vi "Write Forecast and Price Data to Optimization.vi"(6 "Max Forecast Length (-1: no limit)":i32=-1, 7 "Bus by ID":T1[](array[typedef]), 8 "error in":errorcluster, 11 "Generic Optimization in":refnum<class "Generic Optimization.lvclass">) -> (0 "error out":errorcluster, 3 "Generic Optimization out":refnum<class "Generic Optimization.lvclass">)   [LabVIEW 2018, in "Generic Optimization Actor.lvlib" / "Generic Optimization.lvclass"]
uses:
  Generic Optimization.lvclass
  C:/Users/Administrator/Desktop/2018LabVIEW EMS/EMS Generic Actor/EMS Generic/EMS Generic.lvclass
  C:/Users/Administrator/Desktop/2018LabVIEW EMS/Device Communication and Control Abstract Actor/Device Communication and Control Abstract/Device Communication and Control Abstract.lvclass
  Optimization Controls/Bus by ID.ctl
  <vilib>/ORNL/CSEISMIC DDS/CSEISMIC DDS Base/Data Types/Controls/DeviceID.ctl
  EMS Generic Actor/EMS Generic/EMS Generic.lvclass/EMS Generic.ctl
  <vilib>/ORNL/CSEISMIC DDS/CSEISMIC DDS Base/Data Types/Controls/DeviceClass Selector.ctl
  <vilib>/ORNL/CSEISMIC DDS/CSEISMIC DDS Base/Data Types/DER_Info.ctl
  <vilib>/ORNL/CSEISMIC DDS/CSEISMIC DDS Base/Data Types/SmartRelay_Measurement.ctl
  <vilib>/ORNL/CSEISMIC DDS/CSEISMIC DDS Base/Data Types/DER_Measurement.ctl
  <vilib>/ORNL/CSEISMIC DDS/CSEISMIC DDS Base/Data Types/ForecastData_Data.ctl
  <vilib>/ActorFramework/Actor/Actor.lvclass/Actor.ctl
  Device Communication and Control Abstract Actor/Device Communication and Control Abstract/Device Communication and Control Abstract.lvclass/Device Communication and Control Abstract.ctl
  Device Communication and Control Abstract Actor/Device Communication and Control Abstract Messages/Set ForecastData Long Msg/Set ForecastData Long Msg.lvclass/Set ForecastData Long Msg.ctl
  <vilib>/ActorFramework/Message Enqueuer/Message Enqueuer.lvclass/Message Enqueuer.ctl
  Generic Optimization.lvclass/Generic Optimization.ctl
  Device Communication and Control Abstract Actor/Device Communication and Control Abstract Messages/Set ForecastData Long Msg/Send Set ForecastData Long.vi
  <vilib>/ActorFramework/Actor/Read Caller Enqueuer.vi
  <vilib>/ActorFramework/Message Enqueuer/Enqueue.vi
  Device Communication and Control Abstract Actor/Device Communication and Control Abstract/Device Communication and Control Abstract.lvclass
  C:/Program Files (x86)/National Instruments/LabVIEW 2018/vi.lib/ActorFramework/Actor/Actor.lvclass
  Device Communication and Control Abstract Actor/Device Communication and Control Abstract Messages/Set ForecastData Long Msg/Set ForecastData Long Msg.lvclass
  C:/Program Files (x86)/National Instruments/LabVIEW 2018/vi.lib/ActorFramework/Message/Message.lvclass
  <vilib>/ActorFramework/Message Priority Queue/Priority Enqueue.vi
  <vilib>/ORNL/CSEISMIC DDS/CSEISMIC DDS Base/CSEISMIC DDS.lvclass
  EMS Generic Actor/EMS Generic/EMS Generic.lvclass
  Utilities/Status Messaging.llb/Status Messaging.lvlib
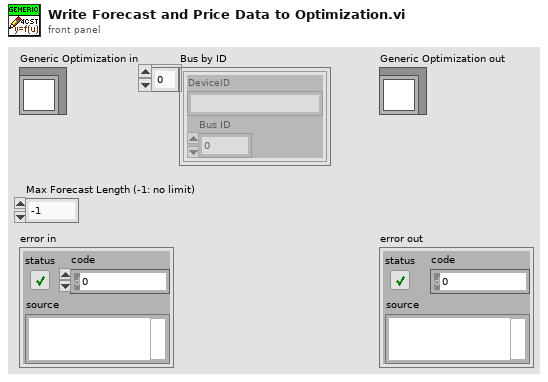
[diagram p1: front panel]
types:
  T1 = typedef "Generic Optimization Actor.lvlib/Generic Optimization.lvclass/Bus by ID.ctl" = cluster{"DeviceID":T2, "Bus ID":dbl}
  T2 = typedef "CSEISMIC DDS.lvlib/CSEISMIC DDS.lvclass/DeviceID.ctl" = string
  T3 = typedef "CSEISMIC DDS.lvlib/CSEISMIC DDS.lvclass/DER_Info.ctl" = cluster{"DeviceID":T2, "LineConfig":u8[], "NominalVoltage(V)":dbl, "PowerRating(kVA)":dbl, "VFControl":bool, "PControl":bool, "QControl":bool, "PFControl":bool, "PVControl":bool, "Droop":bool, "DroopConfigurable":bool, "Unbalanced":bool}
  T4 = typedef "CSEISMIC DDS.lvlib/CSEISMIC DDS.lvclass/ForecastData_Data.ctl" = cluster{"DeviceID":T2, "TargetID":T2, "t0":dbl, "dt":dbl, "Magnitude":dbl[]}
  T5 = typedef "CSEISMIC DDS.lvlib/CSEISMIC DDS.lvclass/SmartRelay_Measurement.ctl" = cluster{"DeviceID":T2, "PrimaryVoltage":dbl[], "SecondaryVoltage":dbl[], "Current":dbl[], "RealPower":dbl[], "ReactivePower":dbl[], "LineConfig":u8[], "Frequency":dbl}
  T6 = typedef "CSEISMIC DDS.lvlib/CSEISMIC DDS.lvclass/DER_Measurement.ctl" = cluster{"DeviceID":T2, "Voltage":dbl[], "Current":dbl[], "RealPower":dbl[], "ReactivePower":dbl[], "LineConfig":u8[], "Frequency":dbl}
  T7 = typedef "EMS Generic Actor.lvlib/EMS Generic.lvclass/Data Type DVRs.ctl" = cluster{"IED_Status":refnum<data-value>, "IED_Status_0":refnum<data-value>, "DER_Measurement":refnum<data-value>, "DER_Info":refnum<data-value>, "DER_Status":refnum<data-value>, "ES_Measurement":refnum<data-value>, "ES_Info":refnum<data-value>, "PV_Info":refnum<data-value>, "SmartRelay_Info":refnum<data-value>, "SmartRelay_Measurement":refnum<data-value>, "Meter_Info":refnum<data-value>, "Meter_Measurement":refnum<data-value>, "HVAC_Status":refnum<data-value>, "HVAC_Measurement":refnum<data-value>, "PriceData_RealTime":refnum<data-value>, "PriceData_Demand":refnum<data-value>, "PriceData_Energy":refnum<data-value>, "ForecastData_Long":refnum<data-value>, "ForecastData_Short":refnum<data-value>, "DER_Control":refnum<data-value>, "DER_SetPointF":refnum<data-value>, "DER_SetPointP":refnum<data-value>, "DER_SetPointQ":refnum<data-value>, "DER_SetPointPF":refnum<data-value>, "DER_SetPointV":refnum<data-value>, "PV_setCurtailment":refnum<data-value>, "PV_setRampRate":refnum<data-value>, "Relay_Control":refnum<data-value>, "Load_Control":refnum<data-value>, "HVAC_Control":refnum<data-value>, "Generator_Info":refnum<data-value>, "ForecastData_Long_Backup":refnum<data-value>, "PriceData_RealTime_Backup":refnum<data-value>}
  T8 = typedef "CSEISMIC DDS.lvlib/CSEISMIC DDS.lvclass/DeviceClass Selector.ctl" = u16
  T9 = typedef "CSEISMIC DDS.lvlib/CSEISMIC DDS.lvclass/PriceData_RealTime.ctl" = cluster{"DeviceID":T2, "t0":dbl, "dt":dbl, "Price":dbl[]}
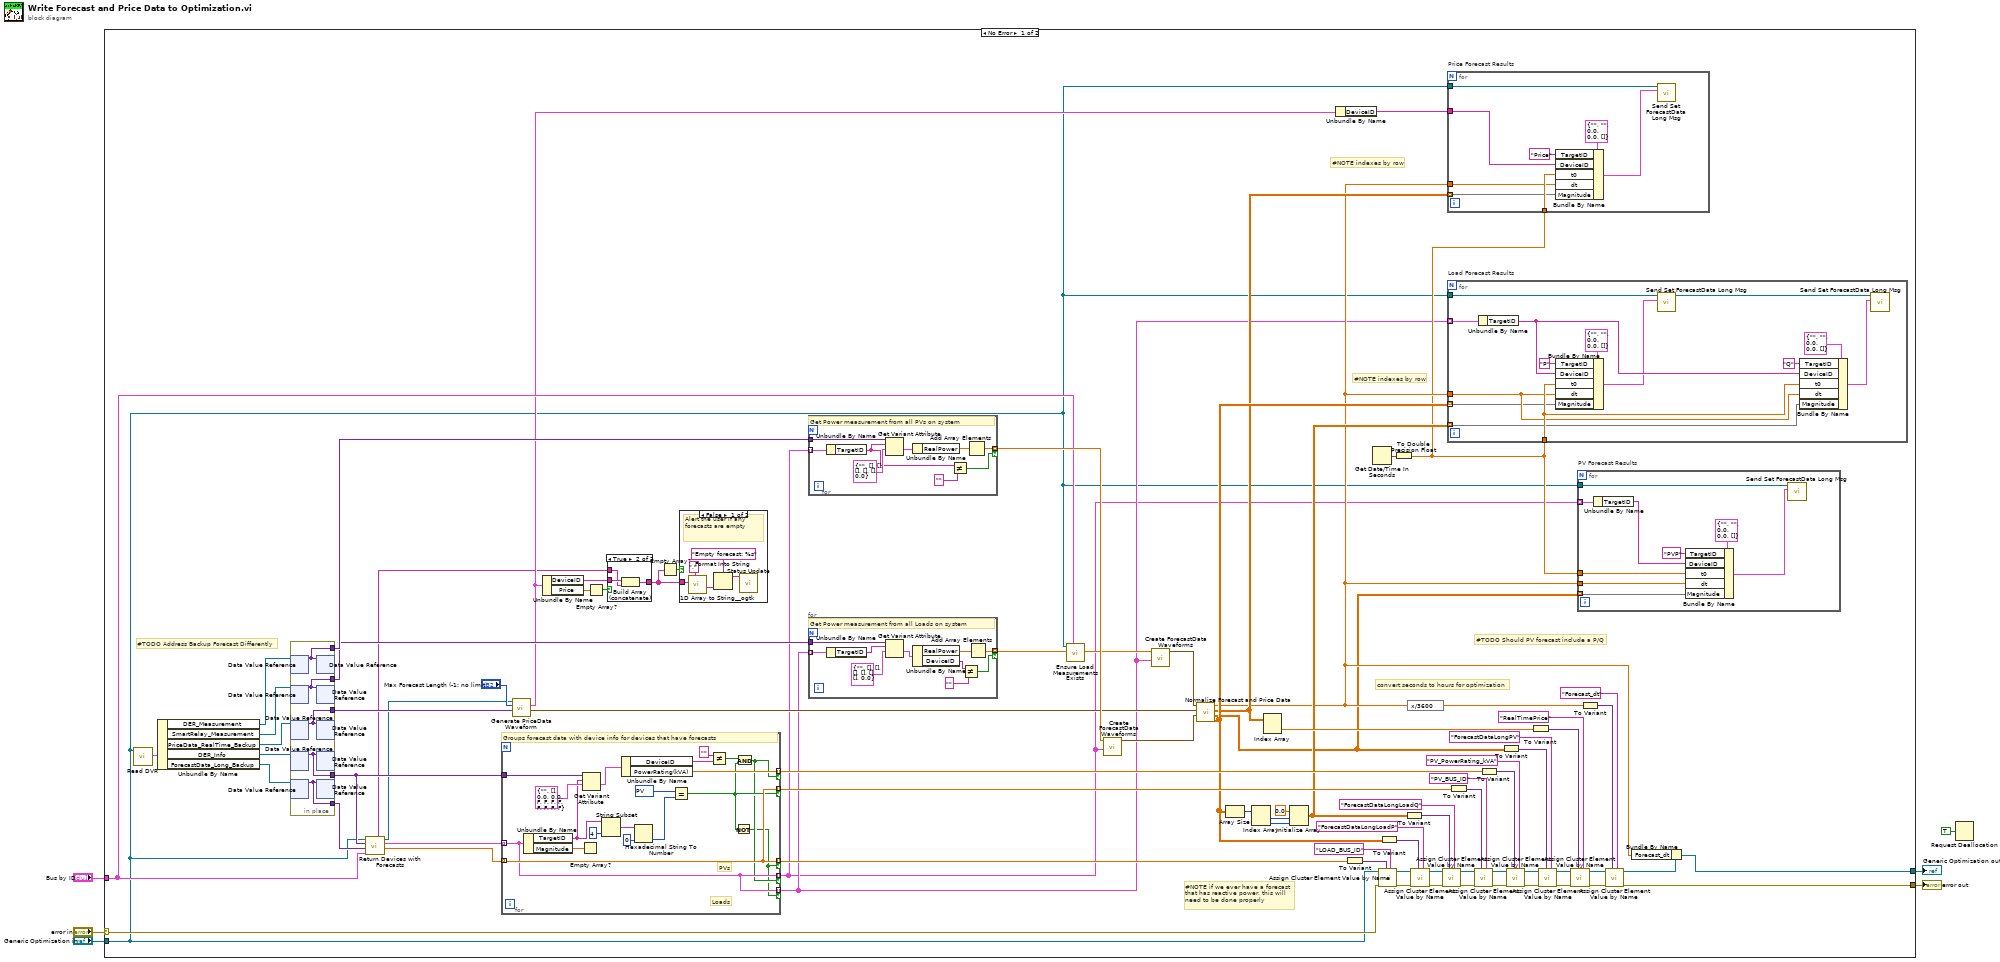
[diagram p0: block diagram]
diagram:
  n1 = case shown="No Error" "error in" {
    selector: "error in" -> [w86 w174]
    tunnel: [w50 w174] -> w5
    tunnel: "Bus by ID" -> [w26 _]
    tunnel: "Generic Optimization in" -> [w9 w173]
    tunnel: [w7 w173] -> w2
    frame No Error {
      # "#NOTE indexes by row"
      # "#NOTE if we ever have a forecast that has reactive power, this will need to be done properly"
      # "#NOTE indexes by row"
      # "convert seconds to hours for optimization"
      # "#TODO Should PV forecast include a P/Q"
      # "#TODO Address Backup Forecast Differently"
      n2 = call "Read DVR.vi"("EMS Generic in"=w9) -> ("DVR"=w59:T7)  [unwired: 9 in, 1 out]
      n3 = Unbundle By Name(w59) -> ("DER_Measurement"=w53:refnum<data-value>, "SmartRelay_Measurement"=w54:refnum<data-value>, "PriceData_RealTime_Backup"=w56:refnum<data-value>, "DER_Info"=w58:refnum<data-value>, "ForecastData_Long_Backup"=w57:refnum<data-value>)
      n4 = in-place {
        in-place-border: [w103] -> w24
        in-place-border: [w102] -> w25
        in-place-border: [w101] -> w22
        in-place-border: [w100] -> w23
        in-place-border: [w99] -> w52
        n5 = in-place-dvr #1(w53) -> (w99:variant)  [unwired: 1 out]
        n6 = in-place-dvr #2(w54) -> (w100:variant)  [unwired: 1 out]
        n7 = in-place-dvr #3(w56) -> (w101:variant)  [unwired: 1 out]
        n8 = in-place-dvr #4(w58) -> (w103:variant)  [unwired: 1 out]
        n9 = in-place-dvr #5(w57) -> (w102:variant)  [unwired: 1 out]
        n10 = in-place-dvr #1(w99) -> ()  [unwired: 2 out]
        n11 = in-place-dvr #2(w100) -> ()  [unwired: 2 out]
        n12 = in-place-dvr #3(w101) -> ()  [unwired: 2 out]
        n13 = in-place-dvr #4(w103) -> ()  [unwired: 2 out]
        n14 = in-place-dvr #5(w102) -> ()  [unwired: 2 out]
      }
      n15 = call "Return Devices with Forecasts.vi"("Bus by ID"=w26, "ForecastData_Long"=w25, "DER_Info"=w24, "Generic Optimization in"=w9) -> ("Device Buses"=w55:dbl[], "Forecasts with Devices"=w27:T4[], "dup Generic Optimization out"=w19:refnum<class "Generic Optimization.lvclass">, "Devices with Empty Forecasts"=w13:T2[])  [unwired: 4 in]
      n16 = for {
        tunnel: w27 -> [w111] mode=indexing
        tunnel: [w117] -> w78 mode=indexing if=w109
        tunnel: [w117] -> w61 mode=indexing if=w112
        tunnel: [w116] -> w60 mode=indexing if=w110
        tunnel: w55 -> [w117] mode=indexing
        tunnel: [w111] -> w17 mode=indexing if=w110
        tunnel: [w111] -> w18 mode=indexing if=w109
        tunnel: w24 -> [w108]
        w119 = T8 514 items=["Invalid"=0, "IED"=256, "DER"=512, "Relay"=768, "Meter"=1024, "Load"=1280, "Forecast"=1536, "Price"=1792, "Energy Storage"=513, "PV"=514, "Generator"=515, "Smart Relay"=769, "PCC"=770, "Smart Meter"=1025, "PMU"=1026, "HVAC"=1281] ("DeviceClass")
        # "PVs"
        # "Loads"
        # "Groups forecast data with device info for devices that have forecasts"
        n17 = Unbundle By Name(w111) -> ("TargetID"=w106:T2, "Magnitude"=w104:dbl[])
        n18 = Empty Array?(array=w104) -> ()  [unwired: 1 out]
        n19 = Get Variant Attribute(Variant=w108, name=w106, default value (empty Variant)=T3 {"DeviceID"="", "LineConfig"=[], "NominalVoltage(V)"=0.0, "PowerRating(kVA)"=0.0, "VFControl"=FALSE, "PControl"=FALSE, "QControl"=FALSE, "PFControl"=FALSE, "PVControl"=FALSE, "Droop"=FALSE, "DroopConfigurable"=FALSE, "Unbalanced"=FALSE} ("DER_Info")) -> (value=w105:T3)  [unwired: 1 in, 3 out]
        n20 = String Subset(string=w106, length (rest)=4 ("length (rest)")) -> (substring=w121:T2)  [unwired: 1 in]
        n21 = Unbundle By Name(w105) -> ("DeviceID"=w113:T2, "PowerRating(kVA)"=w116:dbl)
        n22 = Hexadecimal String To Number(string=w121, default (0uL)=u16 0 ("default (0 U32)")) -> (number=w118:u16)  [unwired: 1 in, 1 out]
        n23 = Equal?(x=w119, y=w118) -> (x = y?=w112:bool)
        n24 = Not Equal?(x=T2 "" ("y"), y=w113) -> (x != y?=w114:bool)
        n25 = Not(x=w112) -> (.not. x?=w109:bool)
        n26 = And(x=w114, y=w112) -> (x .and. y?=w110:bool)
      }
      n27 = call "Generate PriceData Waveform.vi"("PriceData_RealTime_Backup"=w22, "Max Forecast Length"="Max Forecast Length (-1: no limit)", "Generic Optimization in"=w19) -> ("Waveform"=w20:waveform(dbl), "PriceData_RealTime"=w15:T9)  [unwired: 6 in, 1 out]
      n28 = Unbundle By Name(w15) -> ("DeviceID"=w11:T2, "Price"=w14:dbl[])
      n29 = Empty Array?(array=w14) -> (empty?=w12:bool)
      n30 = case shown="True" w12 {
        tunnel: w13 -> [w90 w92]
        tunnel: w11 -> [_ w93]
        tunnel: [w90 w91] -> w10
        frame False {
        }
        frame True {
          n31 = Build Array (concatenate)(w93, w92) -> (w91:T2[])
        }
      }
      n32 = Empty Array?(array=w10) -> (empty?=w16:bool)
      n33 = case shown="False" w16 {
        tunnel: w10 -> [w98 _]
        frame False {
          # "Alert the user if any forecasts are empty"
          n34 = call <userlib>:"1D Array to String__ogtk.vi"("delimiter (Tab)"=",", "Array of Strings"=w98) -> ("delimited string"=w96:string)  [unwired: 9 in]
          n35 = Format Into String(format string="Empty forecast: %s", w96) -> (resulting string=w94:string)  [unwired: 2 in, 1 out]
          n36 = call "Status Update.vi"("Status Update"=w94) -> ()  [unwired: 9 in, 2 out]
        }
        frame True {
        }
      }
      n37 = for {
        tunnel: w17 -> [w172] mode=indexing
        tunnel: w52 -> [w171]
        tunnel: [w167] -> w46 mode=indexing if=w164
        # "Get Power measurement from all PVs on system"
        n38 = Unbundle By Name(w172) -> ("TargetID"=w165:T2)
        n39 = Get Variant Attribute(Variant=w171, name=w165, default value (empty Variant)=T6 {"DeviceID"="", "Voltage"=[], "Current"=[], "RealPower"=[], "ReactivePower"=[], "LineConfig"=[], "Frequency"=0.0} ("DER_Measurement")) -> (value=w169:T6)  [unwired: 1 in, 3 out]
        n40 = Unbundle By Name(w169) -> ("RealPower"=w168:dbl[])
        n41 = Not Equal?(x=w165, y=T2 "") -> (x != y?=w164:bool)
        n42 = Add Array Elements(numeric array=w168) -> (sum=w167:dbl)
      }
      n43 = for {
        tunnel: w18 -> [w163] mode=indexing
        tunnel: w23 -> [w161]
        tunnel: [w158] -> w37 mode=indexing if=w154
        # "Get Power measurement from all Loads on system"
        n44 = Unbundle By Name(w163) -> ("TargetID"=w162:T2)
        n45 = Get Variant Attribute(Variant=w161, name=w162, default value (empty Variant)=T5 {"DeviceID"="", "PrimaryVoltage"=[], "SecondaryVoltage"=[], "Current"=[], "RealPower"=[], "ReactivePower"=[], "LineConfig"=[], "Frequency"=0.0} ("SmartRelay_Measurement")) -> (value=w160:T5)  [unwired: 1 in, 3 out]
        n46 = Unbundle By Name(w160) -> ("RealPower"=w157:dbl[], "DeviceID"=w155:T2)
        n47 = Not Equal?(x=w155, y=T2 "") -> (x != y?=w154:bool)
        n48 = Add Array Elements(numeric array=w157) -> (sum=w158:dbl)
      }
      n49 = call "Ensure Load Measurements Exists.vi"("Bus by ID"=w26, "Load Power Measurements"=w37, "Generic Optimization in"=w9) -> ("Load Power Measurements"=w36:dbl[])  [unwired: 8 in]
      n50 = call "Create ForecastData Waveforms.vi"("ForecastData Array"=w17, "Measured Powers"=w46) -> ("Forecast Waveforms Array"=w44:waveform(dbl)[])  [unwired: 9 in]
      n51 = call "Create ForecastData Waveforms.vi"("ForecastData Array"=w18, "Measured Powers"=w36) -> ("Forecast Waveforms Array"=w45:waveform(dbl)[])  [unwired: 9 in]
      n52 = call "Normalize Forecast and Price Data.vi"("PV Forecast Waveforms Array"=w44, "Price Forecast Waveform"=w20, "Load Forecast Waveforms Array"=w45) -> ("Load Magnitudes"=w33:dbl[][], "PV Magnitudes"=w28:dbl[][], "Price Magnitudes"=w32:dbl[][], "Normalized dt"=w30:dbl)  [unwired: 5 in]
      n53 = Array Size(array=w33) -> (size(s)=w41:i32[])
      n54 = Index Array(array=w41) -> (element #1=w40:i32, element #2=w39:i32)  [unwired: 2 in]
      n55 = Index Array(array=w32) -> (element=w43:dbl[])  [unwired: 2 in]
      n56 = Initialize Array(0.0, w40, w39) -> (w34:dbl[][])
      n57 = Unbundle By Name(w15) -> ("DeviceID"=w31:T2)
      n58 = To Variant(anything=w78) -> (Variant=w85:variant)
      n59 = Get Date/Time In Seconds() -> (seconds since 1Jan1904=w35:timestamp)
      n60 = call "Assign Cluster Element Value by Name.vi"("Element Name"="LOAD_BUS_ID" ("Keyword Name"), "Value"=w85, "error in"=w86, "Generic Optimization"=w9) -> ("error out"=w87:errorcluster, "Generic Optimization out"=w88:refnum<class "Generic Optimization.lvclass">)  [unwired: 6 in]
      n61 = To Variant(anything=w33) -> (Variant=w79:variant)
      n62 = To Double Precision Float(number=w35) -> (double precision float=w29:dbl)
      n63 = To Variant(anything=w34) -> (Variant=w81:variant)
      n64 = expression code="x/3600"(w30) -> (w42:dbl)
      n65 = call "Assign Cluster Element Value by Name.vi"("Element Name"="ForecastDataLongLoadP" ("Keyword Name"), "Value"=w79, "error in"=w87, "Generic Optimization"=w88) -> ("error out"=w84:errorcluster, "Generic Optimization out"=w83:refnum<class "Generic Optimization.lvclass">)  [unwired: 6 in]
      n66 = call "Assign Cluster Element Value by Name.vi"("Element Name"="ForecastDataLongLoadQ" ("Keyword Name"), "Value"=w81, "error in"=w84, "Generic Optimization"=w83) -> ("error out"=w62:errorcluster, "Generic Optimization out"=w63:refnum<class "Generic Optimization.lvclass">)  [unwired: 6 in]
      n67 = for "Price Forecast Results" {
        tunnel: w32 -> [w132] mode=indexing
        tunnel: w29 -> [w137]
        tunnel: w9 -> [w136]
        tunnel: w30 -> [w135]
        tunnel: w31 -> [w134]
        n68 = Bundle By Name(cluster=T4 {"DeviceID"="", "TargetID"="", "t0"=0.0, "dt"=0.0, "Magnitude"=[]} ("ForecastData"), "TargetID"=T2 "Price", "DeviceID"=w134, "t0"=w137, "dt"=w135, "Magnitude"=w132) -> (w133:T4)
        n69 = call "Send Set ForecastData Long Msg.vi"("ForecastData"=w133, "SCADA Sub Abstract in"=w136) -> ()  [unwired: 8 in, 2 out]
      }
      n70 = for "Load Forecast Results" {
        tunnel: w18 -> [w147] mode=indexing
        tunnel: w33 -> [w141] mode=indexing
        tunnel: w34 -> [w140] mode=indexing
        tunnel: w29 -> [w149]
        tunnel: w9 -> [w148]
        tunnel: w30 -> [w145]
        n71 = Unbundle By Name(w147) -> ("TargetID"=w146:T2)
        n72 = Bundle By Name(cluster=T4 {"DeviceID"="", "TargetID"="", "t0"=0.0, "dt"=0.0, "Magnitude"=[]} ("ForecastData"), "TargetID"=T2 "P", "DeviceID"=w146, "t0"=w149, "dt"=w145, "Magnitude"=w141) -> (w143:T4)
        n73 = call "Send Set ForecastData Long Msg.vi"("ForecastData"=w143, "SCADA Sub Abstract in"=w148) -> ("dup SCADA Sub Abstract"=w144:refnum<class "Generic Optimization.lvclass">)  [unwired: 8 in, 1 out]
        n74 = Bundle By Name(cluster=T4 {"DeviceID"="", "TargetID"="", "t0"=0.0, "dt"=0.0, "Magnitude"=[]} ("ForecastData"), "TargetID"=T2 "Q", "DeviceID"=w146, "t0"=w149, "dt"=w145, "Magnitude"=w140) -> (w142:T4)
        n75 = call "Send Set ForecastData Long Msg.vi"("ForecastData"=w142, "SCADA Sub Abstract in"=w144) -> ()  [unwired: 8 in, 2 out]
      }
      n76 = To Variant(anything=w61) -> (Variant=w75:variant)
      n77 = call "Assign Cluster Element Value by Name.vi"("Element Name"="PV_BUS_ID" ("Keyword Name"), "Value"=w75, "error in"=w62, "Generic Optimization"=w63) -> ("error out"=w66:errorcluster, "Generic Optimization out"=w67:refnum<class "Generic Optimization.lvclass">)  [unwired: 6 in]
      n78 = To Variant(anything=w60) -> (Variant=w69:variant)
      n79 = To Variant(anything=w28) -> (Variant=w77:variant)
      n80 = call "Assign Cluster Element Value by Name.vi"("Element Name"="PV_PowerRating_kVA" ("Keyword Name"), "Value"=w69, "error in"=w66, "Generic Optimization"=w67) -> ("error out"=w65:errorcluster, "Generic Optimization out"=w64:refnum<class "Generic Optimization.lvclass">)  [unwired: 6 in]
      n81 = To Variant(anything=w43) -> (Variant=w73:variant)
      n82 = call "Assign Cluster Element Value by Name.vi"("Element Name"="ForecastDataLongPV" ("Keyword Name"), "Value"=w77, "error in"=w65, "Generic Optimization"=w64) -> ("error out"=w70:errorcluster, "Generic Optimization out"=w71:refnum<class "Generic Optimization.lvclass">)  [unwired: 6 in]
      n83 = call "Assign Cluster Element Value by Name.vi"("Element Name"="RealTimePrice" ("Keyword Name"), "Value"=w73, "error in"=w70, "Generic Optimization"=w71) -> ("error out"=w51:errorcluster, "Generic Optimization out"=w49:refnum<class "Generic Optimization.lvclass">)  [unwired: 6 in]
      n84 = for "PV Forecast Results" {
        tunnel: w28 -> [w123] mode=indexing
        tunnel: w9 -> [w129]
        tunnel: w30 -> [w128]
        tunnel: w17 -> [w127] mode=indexing
        tunnel: w29 -> [w125]
        n85 = Unbundle By Name(w127) -> ("TargetID"=w126:T2)
        n86 = Bundle By Name(cluster=T4 {"DeviceID"="", "TargetID"="", "t0"=0.0, "dt"=0.0, "Magnitude"=[]} ("ForecastData"), "TargetID"=T2 "PVP", "DeviceID"=w126, "t0"=w125, "dt"=w128, "Magnitude"=w123) -> (w124:T4)
        n87 = call "Send Set ForecastData Long Msg.vi"("ForecastData"=w124, "SCADA Sub Abstract in"=w129) -> ()  [unwired: 8 in, 2 out]
      }
      n88 = To Variant(anything=w42) -> (Variant=w47:variant)
      n89 = call "Assign Cluster Element Value by Name.vi"("Element Name"="Forecast_dt" ("Keyword Name"), "Value"=w47, "error in"=w51, "Generic Optimization"=w49) -> ("error out"=w50:errorcluster, "Generic Optimization out"=w8:refnum<class "Generic Optimization.lvclass">)  [unwired: 6 in]
      n90 = Bundle By Name(cluster=w8, "Forecast_dt"=w30) -> (w7:refnum<class "Generic Optimization.lvclass">)
    }
    frame Error {
    }
  }
  "error out" <- w5
  "Generic Optimization out" <- w2
  n91 = Request Deallocation(TRUE ("flag")) -> ()
